vi "Initialize.vi"(7 "Serial Configuration":T1={"Baud Rate"=9600, "Flow Control"=0, "Parity"=0, "Data Bits"=8} {"Flow Control" items=["NONE", "SOFTWARE"]; "Data Bits" items=["7"=7, "8"=8]; "Parity" items=["NONE", "ODD", "EVEN"]; "Baud Rate" items=["300"=300, "600"=600, "1200"=1200, "2400"=2400, "4800"=4800, "9600"=9600, "19200"=19200]}, 8 "error in (no error)":errorcluster, 9 "Reset (True)":bool=TRUE, 10 "ID Query (True)":bool=TRUE, 11 "VISA resource name":refnum<visa-resource-name>) -> (0 "error out":errorcluster, 3 "VISA resource name out":refnum<visa-resource-name>)   [LabVIEW 2025]
doc: "Establishes communication with the instrument and optionally performs an instrument identification query and/or an instrument reset. It also places the instrument in a default state needed for other instrument driver operations. Therefore, call this VI before calling other instrument driver VIs for this instrument. Generally, you need to call the <b>Initialize</b> VI only once at the beginning of an application."
uses:
  <vilib>/ErrorRing/Error Ring.xnode
panel:
  # "(c) 2025 <RAMON TABOADA>.  ALL RIGHTS RESERVED."
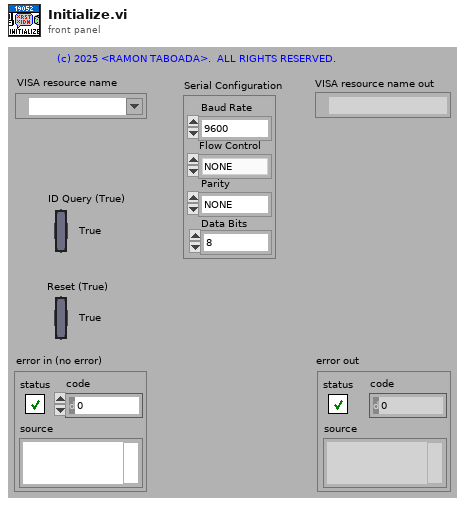
[diagram p1: front panel]
types:
  T1 = cluster{"Baud Rate":u32, "Flow Control":u16, "Parity":u16, "Data Bits":u16}
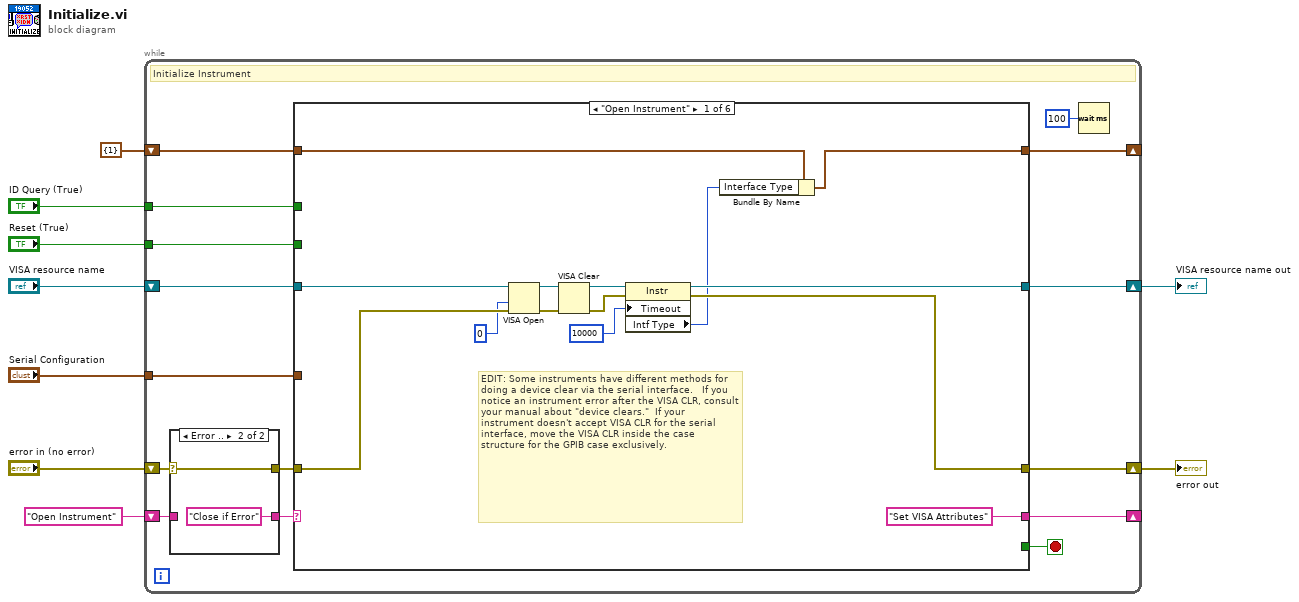
[diagram p0: block diagram]
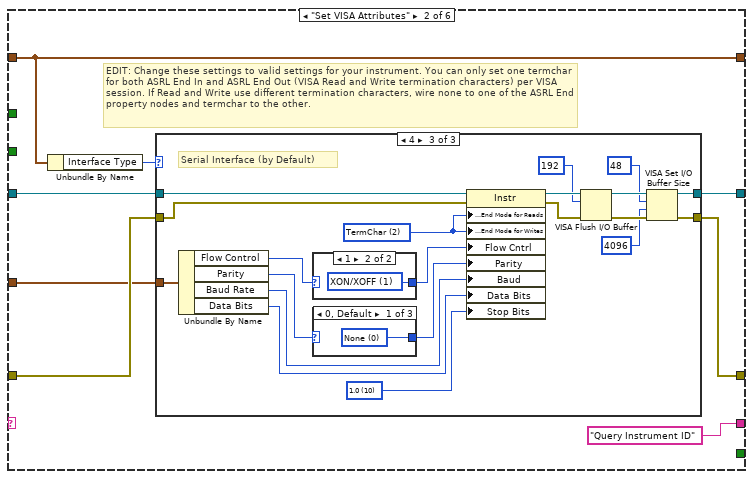
[diagram p3: hidden frame]
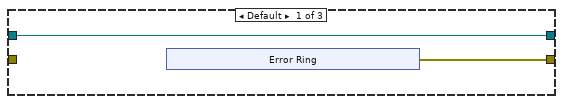
[diagram p4: hidden frame]
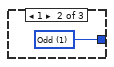
[diagram p6: hidden frame]
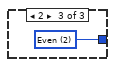
[diagram p7: hidden frame]
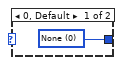
[diagram p8: hidden frame]
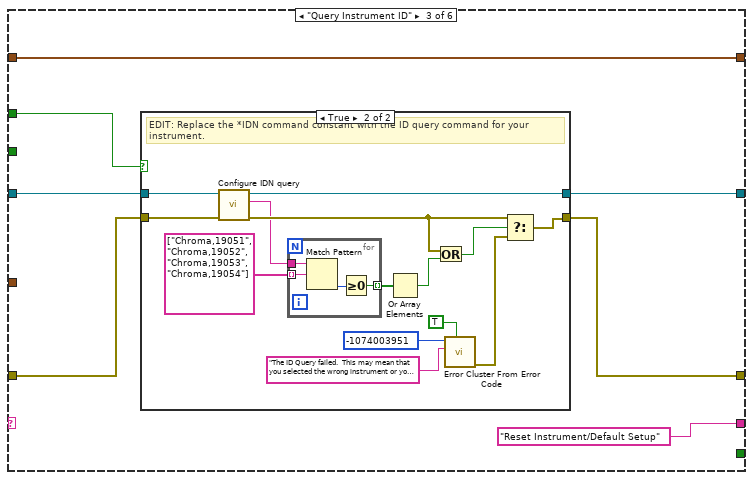
[diagram p9: hidden frame]
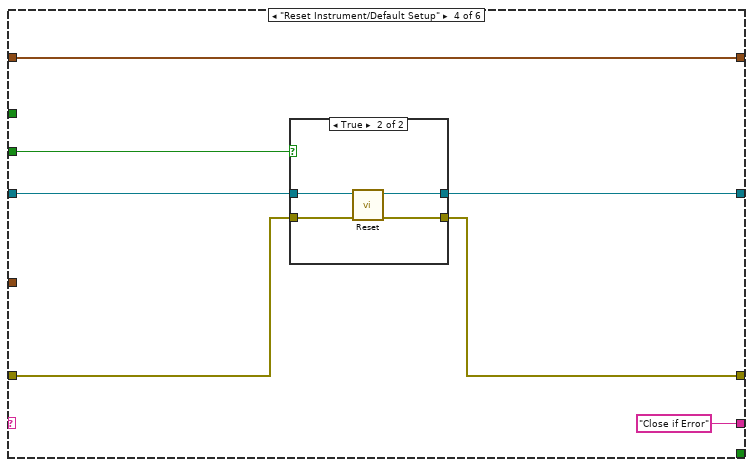
[diagram p11: hidden frame]
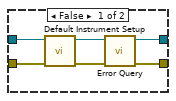
[diagram p12: hidden frame]
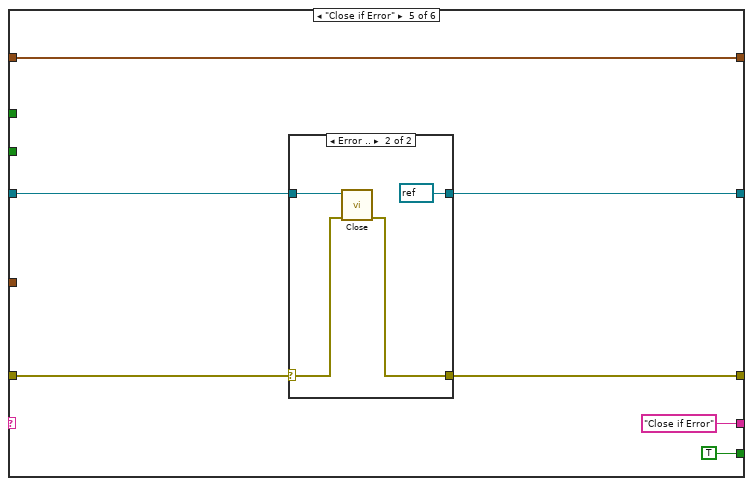
[diagram p13: hidden frame]
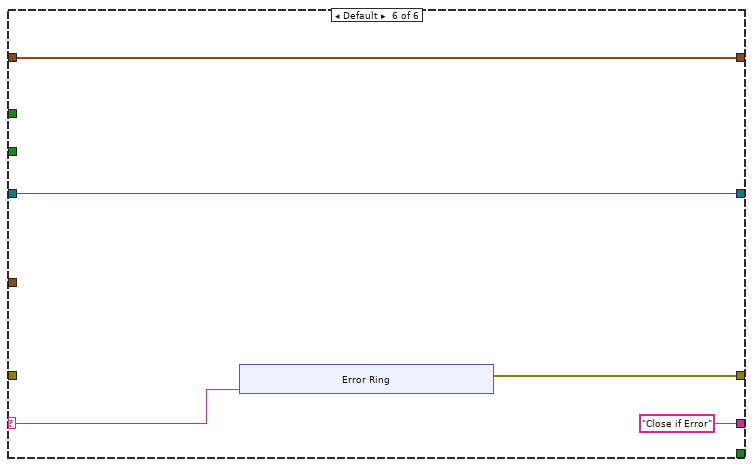
[diagram p15: hidden frame]
diagram:
  n1 = while {
    shift-right: [w23] -> _
    shift-left: cluster{"Interface Type":u16} {"Interface Type"=1} -> [w24]
    shift-right: [w22] -> _
    shift-left: "Open Instrument" -> [w15]
    shift-right: [w21] -> w1
    shift-left: "error in (no error)" -> [w17]
    tunnel: "Reset (True)" -> [w13]
    tunnel: "ID Query (True)" -> [w12]
    tunnel: "Serial Configuration" -> [w11]
    shift-right: [w20] -> w2
    shift-left: "VISA resource name" -> [w19]
    stop <- w18 stop-if-true
    # "Initialize Instrument"
    n2 = case shown="Error .." w17 {
      selector: w17 -> [w26 w28]
      tunnel: [w26 w28] -> w16
      tunnel: w15 -> [w25 _]
      tunnel: [w25 "Close if Error"] -> w14
      frame No Error {
      }
      frame Error {
      }
    }
    n3 = case shown="\"Open Instrument\"" w14 {
      selector: w14 -> [_ _ _ _ _ w144]
      tunnel: w24 -> [w39 w50 w91 w118 w135 w146]
      tunnel: [w38 w50 w91 w118 w135 w146] -> w23
      tunnel: ["Set VISA Attributes" "Query Instrument ID" "Reset Instrument/Default Setup" "Close if Error" "Close if Error" "Close if Error"] -> w22
      tunnel: [w31 w43 w85 w112 w129 w143] -> w21
      tunnel: w16 -> [w40 w49 w89 w117 w132 _]
      tunnel: [w42 w48 w88 w115 w130 w145] -> w20
      tunnel: w19 -> [w35 w46 w90 w116 w131 w145]
      tunnel: [_ _ _ _ TRUE _] -> w18
      tunnel: w13 -> [_ _ _ w113 _ _]
      tunnel: w12 -> [_ _ w86 _ _ _]
      tunnel: w11 -> [_ w45 _ _ _ _]
      frame "Open Instrument" {
        # "EDIT: Some instruments have different methods for doing a device clear via the serial interface.   If you notice an instrument error after the VISA CLR, consult your manual about \"device clears.\"  If your instrument doesn't accept VISA CLR for the serial interface, move the VISA CLR inside the case  structure for the GPIB case exclusively."
        n4 = VISA Open(access mode=u32 0, error in (no error)=w40, VISA resource name=w35) -> (VISA resource name=w41:refnum<visa-resource-name>, error out=w36:errorcluster)  [unwired: 2 in]
        n5 = VISA Clear(VISA resource name=w41, error in (no error)=w36) -> (VISA resource name out=w34:refnum<visa-resource-name>, error out=w33:errorcluster)
        n6 = property class="Instr"(reference=w34, error in=w33, "Timeout"=u32 10000 ("Tmo Value")) -> (reference out=w42:refnum<visa-resource-name>, error out=w31:errorcluster, "Intf Type"=w29:u16)
        n7 = Bundle By Name(cluster=w39, "Interface Type"=w29) -> (w38:cluster{"Interface Type":u16})
      }
      frame "Set VISA Attributes" {
        # "EDIT: Change these settings to valid settings for your instrument. You can only set one termchar for both ASRL End In and ASRL End Out (VISA Read and Write termination characters) per VISA session. If Read and Write use different termination characters, wire none to one of the ASRL End property nodes and termchar to the other."
        n8 = Unbundle By Name(w50) -> ("Interface Type"=w44:u16)
        n9 = case shown="4" w44 {
          tunnel: [w52 w58 w63] -> w48
          tunnel: [w51 w59 w65] -> w43
          tunnel: w49 -> [_ w59 w78]
          tunnel: w46 -> [w52 w58 w79]
          tunnel: w45 -> [_ _ w68]
          frame Default {
            n10 = xnode "Error Ring"() -> ("error out"=w51:errorcluster)
          }
          frame 1 {
            # "GPIB when interface is installed"
          }
          frame 4 {
            w60 = u16 10 items=["1.0"=10, "1.5"=15, "2.0"=20] ("Serial Settings:Stop Bits")
            w76 = u16 2 items=["None", "LastBit", "TermChar"] ("Serial Settings:Serial End Mode for Reads")
            # "Serial Interface (by Default)"
            n11 = Unbundle By Name(w68) -> ("Flow Control"=w75:u16, "Parity"=w74:u16, "Baud Rate"=w72:u32, "Data Bits"=w71:u16)
            n12 = case shown="1" w75 {
              tunnel: [w83 w84] -> w70
              frame 0, Default {
                w83 = u16 0 items=["None", "XON/XOFF", "RTS/CTS", "XON/XOFF & RTS/CTS", "DTR/DSR", "XON/XOFF & DTR/DSR"] ("Serial Settings:Flow Control")
              }
              frame 1 {
                w84 = u16 1 items=["None", "XON/XOFF", "RTS/CTS", "XON/XOFF & RTS/CTS", "DTR/DSR", "XON/XOFF & DTR/DSR"] ("Serial Settings:Flow Control")
              }
            }
            n13 = case shown="0, Default" w74 {
              tunnel: [w80 w81 w82] -> w73
              frame 0, Default {
                w80 = u16 0 items=["None", "Odd", "Even", "Mark", "Space"] ("Serial Settings:Parity")
              }
              frame 1 {
                w81 = u16 1 items=["None", "Odd", "Even", "Mark", "Space"] ("Serial Settings:Parity")
              }
              frame 2 {
                w82 = u16 2 items=["None", "Odd", "Even", "Mark", "Space"] ("Serial Settings:Parity")
              }
            }
            n14 = property class="Instr"(reference=w79, error in=w78, "Serial Settings:End Mode for Reads"=w76, "Serial Settings:End Mode for Writes"=w76, "Flow Cntrl"=w70, "Parity"=w73, "Baud"=w72, "Data Bits"=w71, "Stop Bits"=w60) -> (reference out=w77:refnum<visa-resource-name>, error out=w69:errorcluster)
            n15 = VISA Flush I/O Buffer(VISA resource name=w77, mask (16)=u16 192, error in (no error)=w69) -> (VISA resource name out=w64:refnum<visa-resource-name>, error out=w66:errorcluster)
            n16 = VISA Set I/O Buffer Size(VISA resource name=w64, mask (16)=u16 48, size (4096)=u32 4096, error in (no error)=w66) -> (VISA resource name out=w63:refnum<visa-resource-name>, error out=w65:errorcluster)
          }
        }
      }
      frame "Query Instrument ID" {
        n17 = case shown="True" w86 {
          tunnel: [w92 w107] -> w85
          tunnel: [w93 w94] -> w88
          tunnel: w90 -> [w93 w98]
          tunnel: w89 -> [w92 w97]
          frame False {
          }
          frame True {
            # "EDIT: Replace the *IDN command constant with the ID query command for your instrument."
            n18 = call "Configure IDN query.vi"("error in (no error)"=w97, "VISA resource name"=w98) -> ("error out"=w96:errorcluster, "Result"=w95:string, "VISA resource name out"=w94:refnum<visa-resource-name>)  [unwired: 7 in]
            n19 = for {
              tunnel: string[] ["Chroma,19051", "Chroma,19052", "Chroma,19053", "Chroma,19054"] -> [w108] mode=indexing
              tunnel: w95 -> [w110]
              tunnel: [w109] -> w101 mode=indexing
              n20 = Match Pattern(string=w110, regular expression=w108) -> (offset past match=w111:i32)  [unwired: 1 in, 3 out]
              n21 = Greater Or Equal To 0?(x=w111) -> (x >= 0?=w109:bool)
            }
            n22 = Or Array Elements(Boolean array=w101) -> (logical OR=w100:bool)
            n23 = Or(x=w96, y=w100) -> (x .or. y?=w99:bool)
            n24 = call <vilib>:"Error Cluster From Error Code.vi"("show call chain? (False)"=TRUE, "error message (\"\")"="The ID Query failed.  This may mean that you selected the wrong instrument or your instrument did not respond.  You may also be using a model that is not officially supported by this driver.  If you are sure that you have selected the correct instrument and it is responding, try disabling the ID Query." ("Source (VI Name)"), "error code (0)"=-1074003951 ("Code")) -> ("error out"=w106:errorcluster)  [unwired: 6 in]
            n25 = Select(t=w96, s=w99, f=w106) -> (s? t:f=w107:errorcluster)
          }
        }
      }
      frame "Reset Instrument/Default Setup" {
        n26 = case shown="True" w113 {
          tunnel: w117 -> [w122 w128]
          tunnel: [w119 w127] -> w112
          tunnel: w116 -> [w121 w126]
          tunnel: [w120 w125] -> w115
          frame False {
            n27 = call <instrlib>:"Default Instrument Setup.vi"("error in (no error)"=w122, "VISA resource name"=w121) -> ("error out"=w123:errorcluster, "VISA resource name out"=w124:refnum<visa-resource-name>)  [unwired: 8 in]
            n28 = call "Error Query.vi"("error in (no error)"=w123, "VISA resource name"=w124) -> ("error out"=w119:errorcluster, "VISA resource name out"=w120:refnum<visa-resource-name>)  [unwired: 6 in, 2 out]
          }
          frame True {
            n29 = call "Reset.vi"("error in (no error)"=w128, "VISA resource name"=w126) -> ("error out"=w127:errorcluster, "VISA resource name out"=w125:refnum<visa-resource-name>)  [unwired: 8 in]
          }
        }
      }
      frame "Close if Error" {
        n30 = case shown="Error .." w132 {
          selector: w132 -> [w137 w140]
          tunnel: w131 -> [w136 w138]
          tunnel: [w136 refnum<visa-resource-name> refnum ("VISA resource name")] -> w130
          tunnel: [w137 w139] -> w129
          frame No Error {
          }
          frame Error {
            n31 = call "Close.vi"("error in (no error)"=w140, "VISA resource name"=w138) -> ("error out"=w139:errorcluster)  [unwired: 9 in]
          }
        }
      }
      frame Default {
        n32 = xnode "Error Ring"("parameter 0"=w144) -> ("error out"=w143:errorcluster)
      }
    }
    n33 = Wait (ms)(milliseconds to wait=u32 100) -> ()  [unwired: 1 out]
  }
  "VISA resource name out" <- w2
  "error out" <- w1
